vi "Quadratic Programming AS.vi"(4 "stopping criteria":T1={"function tolerance"=1e-08, "parameter tolerance"=1000000.0, "max iterations"=10000, "max function calls"=10000, "gradient tolerance"=1000000.0, "max time (sec)"=-1.0}, 5 "warm start?":bool, 6 "inequality constraints":cluster{"D":dbl[][], "Imin":dbl[], "Imax":dbl[]}, 7 "start":dbl[](array[numeric]), 8 "error in (no error)":errorcluster, 9 "equality constraints":cluster{"A":dbl[][], "b":dbl[]}, 10 "parameter bounds":cluster{"Xmin":dbl[], "Xmax":dbl[]}, 11 "objective function":cluster{"Q":dbl[][], "c":dbl[]}) -> (0 "error out":errorcluster, 1 "lagrangian multipliers":dbl[](array[numeric]), 2 "f(minimum)":dbl, 3 "minimum":dbl[](array[numeric]))   [LabVIEW 2017, in "NI_Gmath.lvlib"]
doc: "Uses either an interior point algorithm or an active set algorithm to solve the problem: minimize 0.5x*Q*x + c*x, such that A*x=b and <B>Imin</B> are less than or equal to D*x, which is less than or equal to <B>Imax</B>. You must manually select the polymorphic instance to use."
uses:
  <vilib>/gmath/NI_Gmath.lvlib
  <vilib>/gmath/NumericalOptimization/stopping criteria.ctl
  <vilib>/Analysis/baseanly.llb/Unit Vector (DBL).vi
  <vilib>/Analysis/7linalg.llb/Create Special Real Matrix.vi
  <vilib>/Analysis/NI_AALPro.lvlib
  <vilib>/Analysis/NI_AALBase.lvlib
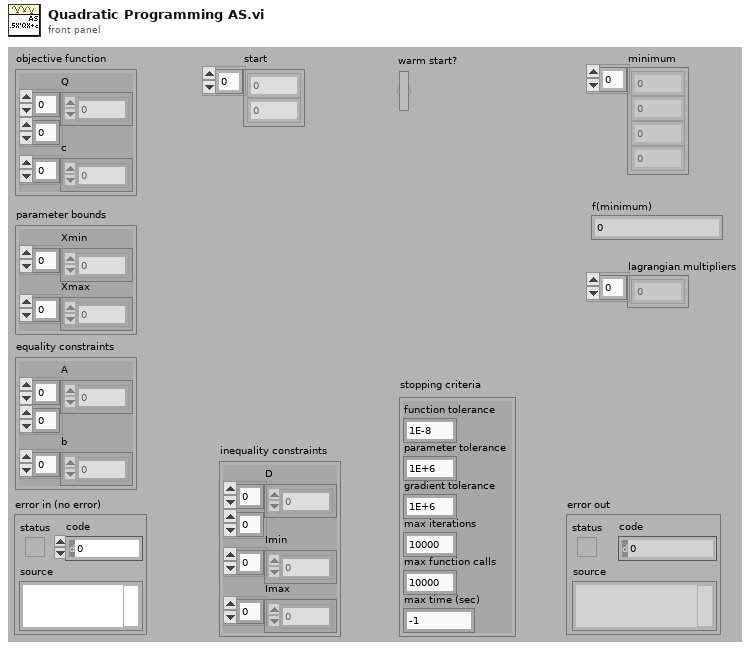
[diagram p1: front panel]
types:
  T1 = typedef "NI_Gmath.lvlib/stopping criteria.ctl" = cluster{"function tolerance":dbl, "parameter tolerance":dbl, "max iterations":i32, "max function calls":i32, "gradient tolerance":dbl, "max time (sec)":dbl}
  T2 = enum32{"Identity", "Diagonal", "Toepliz", "Vandermonde", "Companion"}
  T3 = enum32{"move out of working set", "move into working set", "unchanged working set"}
  T4 = typedef "NI_Gmath.lvlib/stopping criteria with time.ctl" = cluster{"function tolerance":dbl, "parameter tolerance":dbl, "max iterations":i32, "max function calls":i32, "gradient tolerance":dbl, "max time (sec)":dbl, "initial tick count":u32}
  T5 = typedef "NI_Matrix.lvlib/RealMatrix.ctl" = dbl[][]
  T6 = typedef "NI_Gmath.lvlib/qp_problem data.ctl" = cluster{"Q":dbl[][], "c":dbl[], "A":dbl[][], "b":dbl[], "Xmin":dbl[], "Xmax":dbl[], "M":i32, "N":i32, "D":dbl[][], "Imax":dbl[], "Imin":dbl[], "NI":i32, "X":dbl[]}
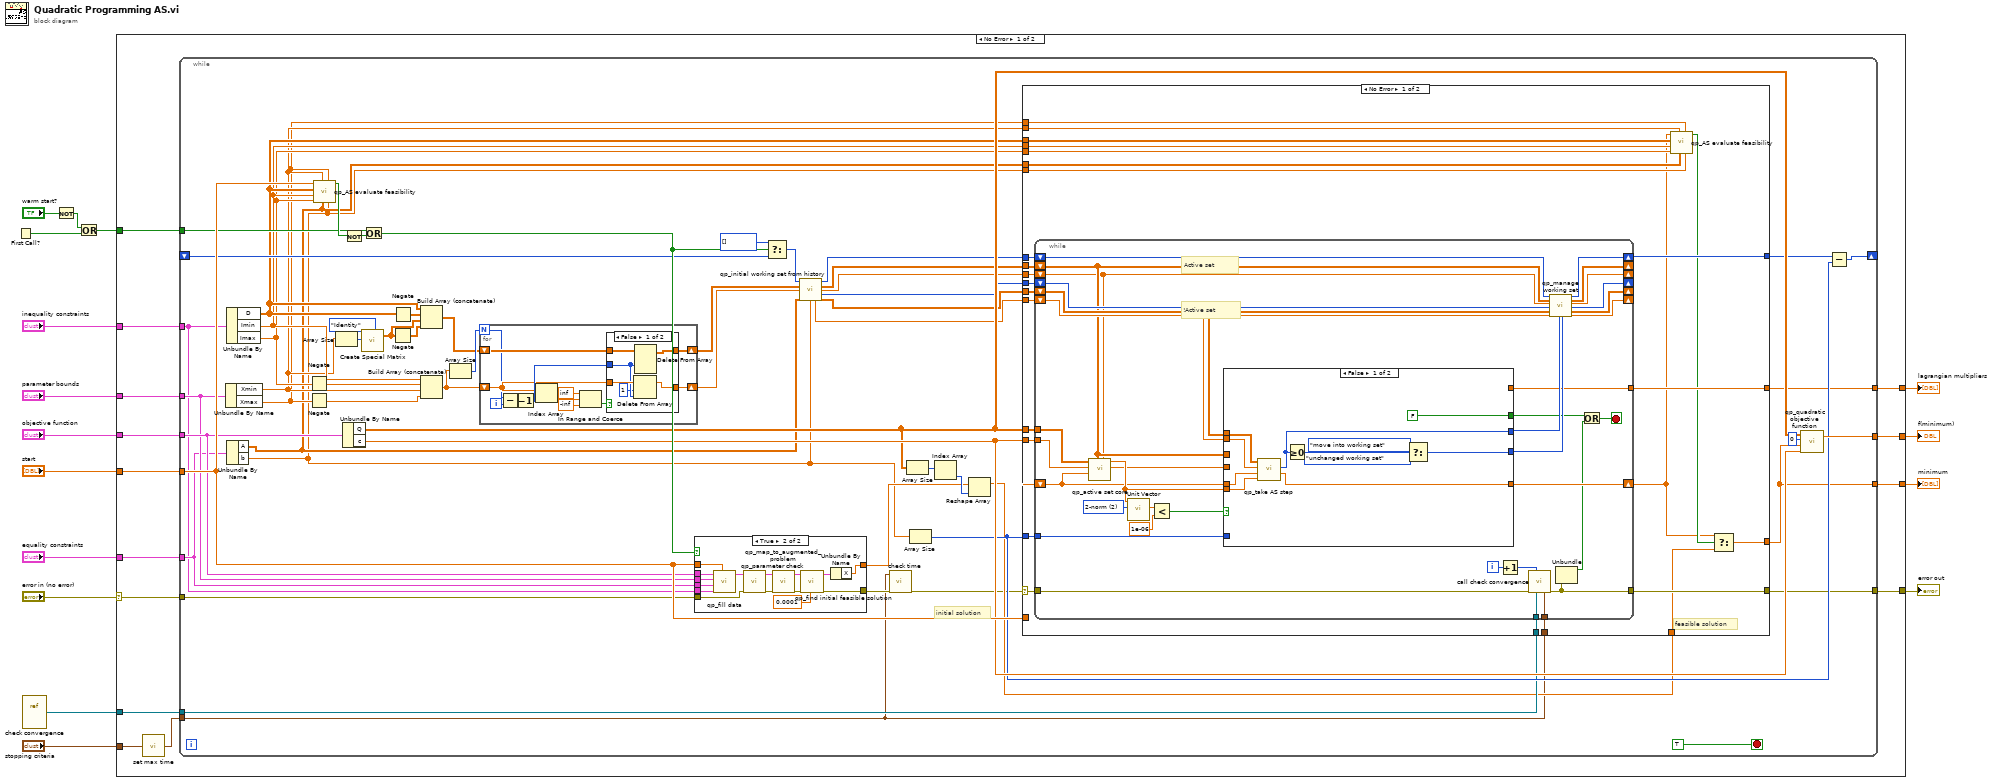
[diagram p0: block diagram]
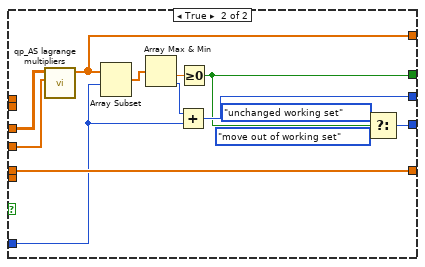
[diagram p3: hidden frame]
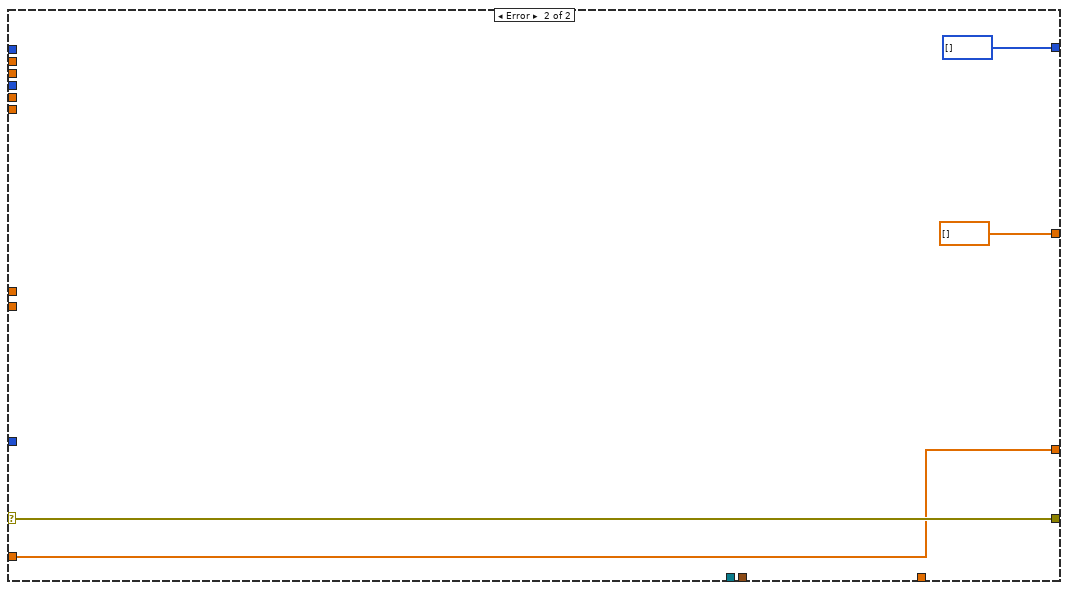
[diagram p4: hidden frame]
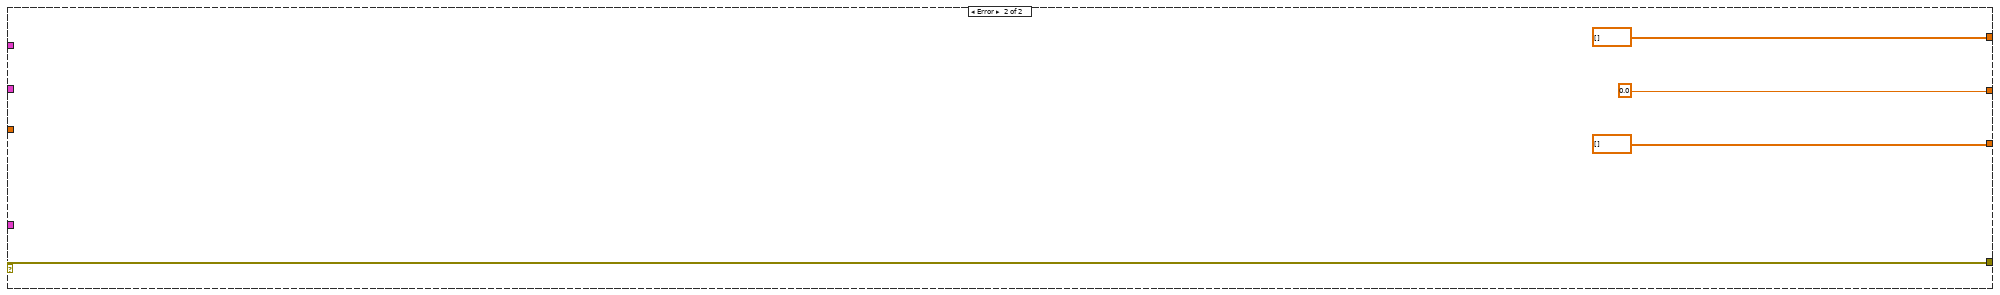
[diagram p6: hidden frame]
diagram:
  n1 = First Call?() -> (First Call?: T/F=w4:bool)
  n2 = vi-ref <vilib>:"check convergence.vi"() -> ("vi reference"=w8:refnum<vi>)
  n3 = Not(x="warm start?") -> (.not. x?=w2:bool)
  n4 = Or(x=w2, y=w4) -> (x .or. y?=w3:bool)
  n5 = case shown="No Error" "error in (no error)" {
    selector: "error in (no error)" -> [w17 w217]
    tunnel: [w30 dbl[] [] ("X")] -> w16
    tunnel: [w29 0.0 ("ob")] -> w15
    tunnel: "objective function" -> [w28 _]
    tunnel: "equality constraints" -> [w27 _]
    tunnel: "parameter bounds" -> [w26 _]
    tunnel: "inequality constraints" -> [w25 _]
    tunnel: "start" -> [w24 _]
    tunnel: [w23 w217] -> w9
    tunnel: w8 -> [w22 _]
    tunnel: [w21 dbl[] [] ("lagrange multipliers")] -> w7
    tunnel: "stopping criteria" -> [w20 _]
    tunnel: w3 -> [w18 _]
    frame No Error {
      n6 = call <vilib>:"set max time.vi"("stopping criteria"=w20) -> ("stopping criteria"=w19:T4)
      n7 = while {
        tunnel: [w33] -> w30
        tunnel: [w79] -> w29
        tunnel: w28 -> [w58]
        tunnel: w27 -> [w56]
        tunnel: w26 -> [w57]
        tunnel: w25 -> [w55]
        tunnel: w24 -> [w87]
        shift-right: [w68] -> _
        shift-left: _ -> [w45]
        tunnel: w18 -> [w44]
        tunnel: [w35] -> w23
        tunnel: w22 -> [w66]
        tunnel: w19 -> [w31]
        tunnel: [w64] -> w21
        tunnel: w17 -> [w50]
        stop <- TRUE stop-if-true
        # "initial solution"
        n8 = Unbundle By Name(w57) -> ("Xmin"=w39:dbl[], "Xmax"=w38:dbl[])
        n9 = Unbundle By Name(w55) -> ("D"=w42:dbl[][], "Imin"=w41:dbl[], "Imax"=w40:dbl[])
        n10 = Unbundle By Name(w56) -> ("A"=w37:dbl[][], "b"=w36:dbl[])
        n11 = Negate(x=w40) -> (-x=w73:dbl[])
        n12 = Negate(x=w38) -> (-x=w83:dbl[])
        n13 = call <vilib>:"qp_AS evaluate feasibility.vi"("b"=w36, "Xmax"=w38, "A"=w37, "Xmin"=w39, "Imax"=w40, "Imin"=w41, "D"=w42, "X"=w87) -> ("feasible?"=w52:bool)  [unwired: 3 in]
        n14 = Array Size(array=w39) -> (size(s)=w84:i32)
        n15 = Unbundle By Name(w58) -> ("Q"=w76:dbl[][], "c"=w81:dbl[])
        n16 = Not(x=w52) -> (.not. x?=w51:bool)
        n17 = call-poly <vilib>:"Create Special Matrix.vi"("matrix type"=T2."Identity", "matrix size"=w84) -> ("Special Matrix"=w75:T5)  [unwired: 3 in, 1 out]
        n18 = Or(x=w44, y=w51) -> (x .or. y?=w86:bool)
        n19 = Negate(x=w75) -> (-x=w74:T5)
        n20 = Negate(x=w42) -> (-x=w85:dbl[][])
        n21 = Build Array (concatenate)(w42, w85, w75, w74) -> (w49:T5)
        n22 = Build Array (concatenate)(w41, w73, w39, w83) -> (w72:dbl[])
        n23 = Array Size(array=w72) -> (size(s)=w82:i32)
        n24 = for {
          N: w82 -> [w196]
          shift-right: [w202] -> w48
          shift-left: w49 -> [w203]
          shift-right: [w201] -> w47
          shift-left: w72 -> [w204]
          i -> [w195]
          n25 = Subtract(x=w196, y=w195) -> (x-y=w194:i32)
          n26 = Decrement(x=w194) -> (x-1=w205:i32)
          n27 = Index Array(array=w204, index=w205) -> (element=w199:dbl)
          n28 = In Range and Coerce(upper limit=inf, x=w199, lower limit=-inf) -> (In Range?=w200:bool)  [unwired: 1 out]
          n29 = case shown="False" w200 {
            tunnel: w205 -> [w207 _]
            tunnel: w204 -> [w209 w212]
            tunnel: w203 -> [w211 w213]
            tunnel: [w210 w213] -> w202
            tunnel: [w208 w212] -> w201
            frame False {
              n30 = Delete From Array(array=w209, length=1, index=w207) -> (array with subset deleted=w208:dbl[])  [unwired: 1 out]
              n31 = Delete From Array(array=w211, index (row)=w207) -> (array with subset deleted=w210:T5)  [unwired: 2 in, 1 out]
            }
            frame True {
            }
          }
        }
        n32 = case shown="True" w86 {
          tunnel: [w88 w104] -> w65
          tunnel: w58 -> [_ w103]
          tunnel: w57 -> [_ w102]
          tunnel: w56 -> [_ w101]
          tunnel: w55 -> [_ w100]
          tunnel: [w89 w92] -> w53
          tunnel: w87 -> [w89 w91]
          tunnel: w50 -> [w88 w90]
          frame False {
          }
          frame True {
            n33 = call <vilib>:"qp_fill data.vi"("x0"=w91, "inequality constraints"=w100, "equality constraints"=w101, "parameter bounds"=w102, "objective function"=w103) -> ("qp data in"=w99:T6)  [unwired: 6 in]
            n34 = call <vilib>:"qp_parameter check.vi"("error in (no error)"=w90, "qp data in"=w99) -> ("error out"=w98:errorcluster, "qp data in"=w95:T6)  [unwired: 8 in]
            n35 = call <vilib>:"qp_map_to_augmented_problem.vi"("error in (no error)"=w98, "qp data in"=w95) -> ("error out"=w97:errorcluster, "qp data out"=w96:T6)  [unwired: 6 in, 2 out]
            n36 = call <vilib>:"qp_find initial feasible solution.vi"("tolerance"=0.0001, "error in (no error)"=w97, "qp data in"=w96) -> ("error out"=w104:errorcluster, "qp data in"=w94:T6)  [unwired: 7 in]
            n37 = Unbundle By Name(w94) -> ("X"=w92:dbl[])
          }
        }
        n38 = Select(t=i32[] [], s=w86, f=w45) -> (s? t:f=w54:i32[])
        n39 = call <vilib>:"qp_initial working set from history.vi"("previous working set indices"=w54, "inequalities"=w48, "inequality constants"=w47, "A"=w37, "b"=w36) -> ("current working set indices"=w63:i32[], "A working set"=w46:T5, "b working set"=w62:dbl[], "not working set indices out"=w61:i32[], "b not working set"=w59:dbl[], "A not working set"=w60:T5)  [unwired: 5 in]
        n40 = call <vilib>:"check time.vi"("error in (no error)"=w65, "stopping criteria"=w31) -> ("error out"=w32:errorcluster)  [unwired: 9 in]
        n41 = Array Size(array=w76) -> (size(s)=w78:i32[])
        n42 = Array Size(array=w36) -> (size(s)=w67:i32)
        n43 = Index Array(array=w78) -> (element=w77:i32)  [unwired: 1 in]
        n44 = Reshape Array(w53, w77) -> (w34:dbl[])
        n45 = case shown="No Error" w32 {
          selector: w32 -> [w109 w193]
          tunnel: w81 -> [w130 _]
          tunnel: w76 -> [w129 _]
          tunnel: [w128 i32[] [] ("current working set indices")] -> w69
          tunnel: w67 -> [w127 _]
          tunnel: w31 -> [w126 _]
          tunnel: w66 -> [w125 _]
          tunnel: [w124 dbl[] [] ("lagrange multipliers")] -> w64
          tunnel: w63 -> [w123 _]
          tunnel: w62 -> [w122 _]
          tunnel: w61 -> [w121 _]
          tunnel: w60 -> [w120 _]
          tunnel: w59 -> [w119 _]
          tunnel: w46 -> [w118 _]
          tunnel: w42 -> [w117 _]
          tunnel: w41 -> [w116 _]
          tunnel: w40 -> [w115 _]
          tunnel: w39 -> [w114 _]
          tunnel: w38 -> [w113 _]
          tunnel: w37 -> [w112 _]
          tunnel: w36 -> [w111 _]
          tunnel: [w110 w193] -> w35
          tunnel: w34 -> [w106 _]
          tunnel: [w105 w190] -> w33
          tunnel: w87 -> [_ w190]
          frame No Error {
            # "feasible solution"
            n46 = while {
              shift-right: [w155] -> w107
              shift-left: w106 -> [w152]
              shift-right: [w143] -> w128
              shift-left: w123 -> [w142]
              tunnel: w129 -> [w161]
              tunnel: w130 -> [w154]
              shift-right: [w165] -> _
              shift-left: w118 -> [w141]
              shift-right: [w164] -> _
              shift-left: w122 -> [w140]
              shift-right: [w163] -> _
              shift-left: w120 -> [w147]
              shift-right: [w162] -> _
              shift-left: w119 -> [w146]
              tunnel: w127 -> [w150]
              shift-right: [w144] -> _
              shift-left: w121 -> [w145]
              tunnel: w109 -> [w132]
              tunnel: [w133] -> w110
              tunnel: w125 -> [w135]
              tunnel: w126 -> [w134]
              tunnel: [w131] -> w124
              i -> [w149]
              stop <- w138 stop-if-true
              w151 = u16 2 items=["1-norm"=1, "2-norm"=2, "Inf-norm"=3, "-Inf-norm"=4, "User Defined"=5] ("norm type")
              # "!Active set"
              # "Active set"
              n47 = call <vilib>:"qp_active set core.vi"("b"=w140, "A"=w141, "x"=w152, "c"=w154, "Q"=w161) -> ("Qx+c"=w153:dbl[], "p_k"=w158:dbl[])  [unwired: 5 in]
              n48 = call-poly <vilib>:"Unit Vector.vi"("norm type"=w151, "Input Vector"=w158) -> ("norm"=w160:dbl)  [unwired: 7 in, 2 out]
              n49 = Less?(x=w160, y=1e-06) -> (x < y?=w148:bool)
              n50 = case shown="False" w148 {
                tunnel: w153 -> [_ w189]
                tunnel: w141 -> [_ w188]
                tunnel: w147 -> [w176 _]
                tunnel: w146 -> [w175 _]
                tunnel: w158 -> [w174 _]
                tunnel: w152 -> [w173 w186]
                tunnel: [FALSE w178] -> w137
                tunnel: [w172 w179] -> w157
                tunnel: [w168 w177] -> w156
                tunnel: [w166 w186] -> w155
                tunnel: w150 -> [_ w183]
                tunnel: [_ w182] -> w131
                frame False {
                  n51 = call <vilib>:"qp_take AS step.vi"("P(k)"=w174, "X(k)"=w173, "b not working set"=w175, "A not working set"=w176) -> ("X(k+1)"=w166:dbl[], "blocking index"=w172:i32)  [unwired: 5 in, 1 out]
                  n52 = Greater Or Equal To 0?(x=w172) -> (x >= 0?=w170:bool)
                  n53 = Select(t=T3."move into working set" ("direction"), s=w170, f=T3."unchanged working set" ("direction")) -> (s? t:f=w168:T3)
                }
                frame True {
                  n54 = call <vilib>:"qp_AS lagrange multipliers.vi"("Qx+c"=w189, "A working set"=w188) -> ("lagrange multipliers"=w182:dbl[])  [unwired: 9 in]
                  n55 = Array Subset(array=w182, index=w183) -> (w184:dbl[])  [unwired: 1 in]
                  n56 = Array Max & Min(array=w184) -> (min value=w187:dbl, min index (indices)=w185:i32)  [unwired: 2 out]
                  n57 = Add(x=w185, y=w183) -> (x+y=w179:i32)
                  n58 = Greater Or Equal To 0?(x=w187) -> (x >= 0?=w178:bool)
                  n59 = Select(t=T3."unchanged working set" ("direction"), s=w178, f=T3."move out of working set" ("direction")) -> (s? t:f=w177:T3)
                }
              }
              n60 = Increment(x=w149) -> (x+1=w136:i32)
              n61 = call <vilib>:"call check convergence.vi"("current iteration"=w136, "error in"=w132, "vi reference"=w135, "stopping criteria"=w134) -> ("error out"=w133:errorcluster)  [unwired: 7 in, 4 out]
              n62 = call <vilib>:"qp_manage working set.vi"("working set indices in"=w142, "A working set"=w141, "b working set"=w140, "not working set indices in"=w145, "A not working set"=w147, "b not working set"=w146, "index"=w157, "direction"=w156) -> ("working set indices out"=w143:i32[], "A working set"=w165:T5, "b working set"=w164:dbl[], "not working set indices out"=w144:i32[], "A not working set"=w163:T5, "b not working set"=w162:dbl[])  [unwired: 6 in]
              n63 = Unbundle(w133) -> ("status"=w139:bool)  [unwired: 2 out]
              n64 = Or(x=w137, y=w139) -> (x .or. y?=w138:bool)
            }
            n65 = call <vilib>:"qp_AS evaluate feasibility.vi"("b"=w111, "Xmax"=w113, "A"=w112, "Xmin"=w114, "Imax"=w115, "Imin"=w116, "D"=w117, "X"=w107) -> ("feasible?"=w108:bool)  [unwired: 3 in]
            n66 = Select(t=w107, s=w108, f=w106) -> (s? t:f=w105:dbl[])
          }
          frame Error {
          }
        }
        n67 = call <vilib>:"qp_quadratic objective function.vi"("c"=w81, "X"=w33, "NI"=0, "Q"=w76) -> ("ob"=w79:dbl)  [unwired: 1 in]
        n68 = Subtract(x=w69, y=w67) -> (x-y=w68:i32[])
      }
    }
    frame Error {
    }
  }
  "minimum" <- w16
  "f(minimum)" <- w15
  "error out" <- w9
  "lagrangian multipliers" <- w7
